vi "test 1.vi"() -> ()   [LabVIEW 2021]
panel:
  out "Tank":dbl(slide) scale=0.0..10.0
  out "Numeric 2":dbl
  in  "Numeric":dbl
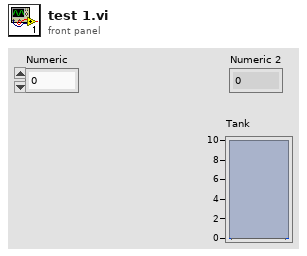
[diagram p1: front panel]
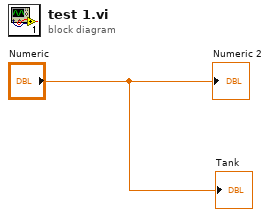
[diagram p0: block diagram]
diagram:
  "Numeric 2" <- "Numeric"
  "Tank" <- "Numeric"
